vi "Loki Not Available Error Constant.vi"(1 "loki url":string) -> (0 "Logger Not Initialized Error":errorcluster)   [LabVIEW 2017, in "hse-logger.lvlib" / "LokiHandler.lvclass"]
uses:
  LokiHandler.lvclass
  LokiHandler.lvclass/LokiHandler.ctl
panel:
  # "Connector Pane"
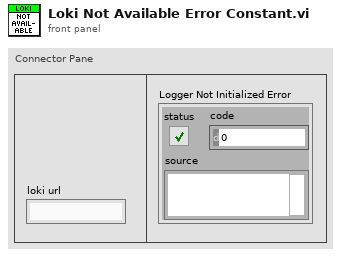
[diagram p1: front panel]
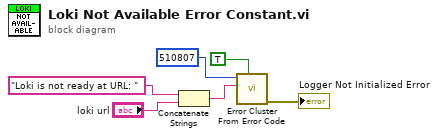
[diagram p0: block diagram]
diagram:
  n1 = Concatenate Strings("Loki is not ready at URL: " ("error message (\"\")"), "loki url") -> (w2:string)
  n2 = call <vilib>:"Error Cluster From Error Code.vi"("show call chain? (False)"=TRUE, "error message (\"\")"=w2, "error code (0)"=510807) -> ("error out"=→"Logger Not Initialized Error":errorcluster)  [unwired: 6 in]
